vi "Set ni_measurementlink_measurement_v1_GetMetadataResponse.vi"(7 "Complete Call (T)":bool=TRUE, 8 "error in (no error)":errorcluster, 10 "package_templatemessage":T1, 11 "gRPCid":T10) -> (0 "error out":errorcluster)   [LabVIEW 2020, in "MeasurementLink Measurement Server Internal.lvlib"]
uses:
  MeasurementLink Measurement Server Internal.lvlib
  <vilib>/gRPC/LabVIEW gRPC Library/Shared/grpcId.ctl
  ni_measurementlink_measurement_v1_GetMetadataResponse.ctl
  ni_measurementlink_measurement_v1_MeasurementDetails.ctl
  ni_measurementlink_measurement_v1_MeasurementSignature.ctl
  ni_measurementlink_measurement_v1_ConfigurationParameter.ctl
  google_protobuf_Field_Kind.ctl
  ni_measurementlink_measurement_v1_ConfigurationParameter_AnnotationsEntry.ctl
  google_protobuf_Any.ctl
  ni_measurementlink_measurement_v1_Output.ctl
  ni_measurementlink_measurement_v1_UserInterfaceDetails.ctl
  ni_measurementlink_measurement_v1_GetMetadataResponse_Flat.ctl
  ni_measurementlink_measurement_v1_MeasurementDetails_Flat.ctl
  ni_measurementlink_measurement_v1_MeasurementSignature_Flat.ctl
  ni_measurementlink_measurement_v1_ConfigurationParameter_Flat.ctl
  ni_measurementlink_measurement_v1_ConfigurationParameter_AnnotationsEntry_Flat.ctl
  google_protobuf_Any_Flat.ctl
  ni_measurementlink_measurement_v1_Output_Flat.ctl
  ni_measurementlink_measurement_v1_UserInterfaceDetails_Flat.ctl
  dcc74a39-081a-4bdd-860b-8ed792803c96.vi
  RichToFlatni_measurementlink_measurement_v1_MeasurementDetails.vi
  RichToFlatni_measurementlink_measurement_v1_MeasurementSignature.vi
  RichToFlatni_measurementlink_measurement_v1_UserInterfaceDetails.vi
  <vilib>/gRPC/LabVIEW gRPC Library/Shared/TranslateGrpcError.vi
  RichToFlatni_measurementlink_measurement_v1_ConfigurationParameter.vi
  RichToFlatgoogle_protobuf_Any.vi
  RichToFlatni_measurementlink_measurement_v1_Output.vi
  RichToFlatni_measurementlink_measurement_v1_ConfigurationParameter_AnnotationsEntry.vi
  <vilib>/gRPC/LabVIEW gRPC Library/Server API/Server/Get Server DLL Path.vi
  <vilib>/Utility/error.llb/Error Cluster From Error Code.vi
  <vilib>/Utility/error.llb/Simple Error Handler.vi
  <vilib>/gRPC/LabVIEW gRPC Library/grpc-lvsupport-release.lvlib
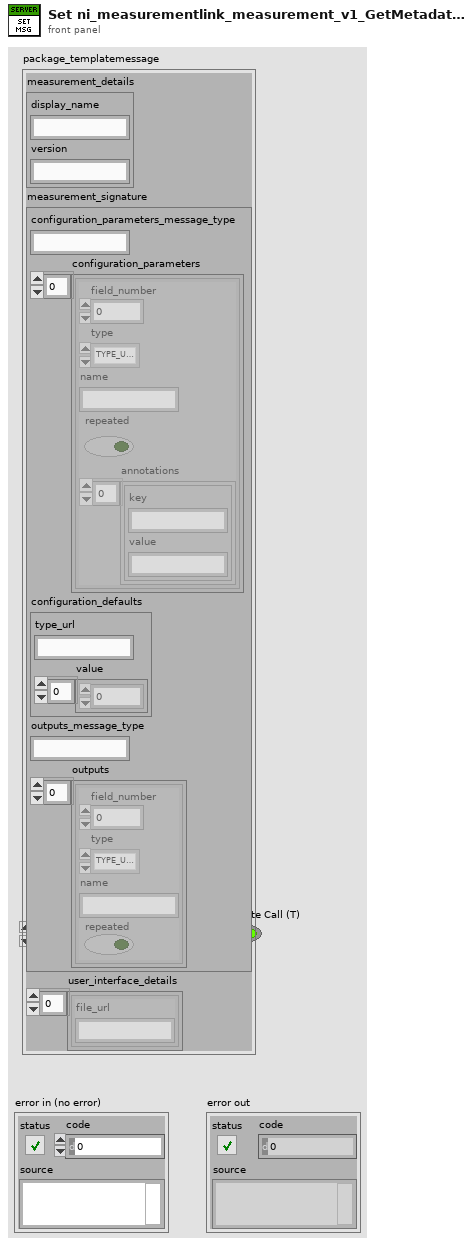
[diagram p1: front panel]
types:
  T1 = typedef "MeasurementLink Measurement Server Internal.lvlib/ni_measurementlink_measurement_v1_GetMetadataResponse.ctl" = cluster{"measurement_details":T2, "measurement_signature":T3, "user_interface_details":T9[]}
  T2 = typedef "MeasurementLink Measurement Server Internal.lvlib/ni_measurementlink_measurement_v1_MeasurementDetails.ctl" = cluster{"display_name":string, "version":string}
  T3 = typedef "MeasurementLink Measurement Server Internal.lvlib/ni_measurementlink_measurement_v1_MeasurementSignature.ctl" = cluster{"configuration_parameters_message_type":string, "configuration_parameters":T4[], "configuration_defaults":T7, "outputs_message_type":string, "outputs":T8[]}
  T4 = typedef "MeasurementLink Measurement Server Internal.lvlib/ni_measurementlink_measurement_v1_ConfigurationParameter.ctl" = cluster{"field_number":i32, "type":T5, "name":string, "repeated":bool, "annotations":T6[]}
  T5 = typedef "MeasurementLink Measurement Server Internal.lvlib/google_protobuf_Field_Kind.ctl" = enum32{"TYPE_UNKNOWN", "TYPE_DOUBLE", "TYPE_FLOAT", "TYPE_INT64", "TYPE_UINT64", "TYPE_INT32", "TYPE_FIXED64", "TYPE_FIXED32", "TYPE_BOOL", "TYPE_STRING", "TYPE_GROUP", "TYPE_MESSAGE", "TYPE_BYTES", "TYPE_UINT32", "TYPE_ENUM", "TYPE_SFIXED32", "TYPE_SFIXED64", "TYPE_SINT32", "TYPE_SINT64"}
  T6 = typedef "MeasurementLink Measurement Server Internal.lvlib/ni_measurementlink_measurement_v1_ConfigurationParameter_AnnotationsEntry.ctl" = cluster{"key":string, "value":string}
  T7 = typedef "MeasurementLink Measurement Server Internal.lvlib/google_protobuf_Any.ctl" = cluster{"type_url":string, "value":u8[]}
  T8 = typedef "MeasurementLink Measurement Server Internal.lvlib/ni_measurementlink_measurement_v1_Output.ctl" = cluster{"field_number":i32, "type":T5, "name":string, "repeated":bool}
  T9 = typedef "MeasurementLink Measurement Server Internal.lvlib/ni_measurementlink_measurement_v1_UserInterfaceDetails.ctl" = cluster{"file_url":string}
  T10 = typedef "grpc-lvsupport-release.lvlib/grpcId.ctl" = u64
  T11 = typedef "MeasurementLink Measurement Server Internal.lvlib/ni_measurementlink_measurement_v1_GetMetadataResponse_Flat.ctl" = cluster{"measurement_details":T12, "measurement_signature":T13, "user_interface_details":T18[]}
  T12 = typedef "MeasurementLink Measurement Server Internal.lvlib/ni_measurementlink_measurement_v1_MeasurementDetails_Flat.ctl" = cluster{"display_name":string, "version":string}
  T13 = typedef "MeasurementLink Measurement Server Internal.lvlib/ni_measurementlink_measurement_v1_MeasurementSignature_Flat.ctl" = cluster{"configuration_parameters_message_type":string, "configuration_parameters":T14[], "configuration_defaults":T16, "outputs_message_type":string, "outputs":T17[]}
  T14 = typedef "MeasurementLink Measurement Server Internal.lvlib/ni_measurementlink_measurement_v1_ConfigurationParameter_Flat.ctl" = cluster{"field_number":i32, "type":T5, "name":string, "repeated":bool, "annotations":T15[]}
  T15 = typedef "MeasurementLink Measurement Server Internal.lvlib/ni_measurementlink_measurement_v1_ConfigurationParameter_AnnotationsEntry_Flat.ctl" = cluster{"key":string, "value":string}
  T16 = typedef "MeasurementLink Measurement Server Internal.lvlib/google_protobuf_Any_Flat.ctl" = cluster{"type_url":string, "value":u8[]}
  T17 = typedef "MeasurementLink Measurement Server Internal.lvlib/ni_measurementlink_measurement_v1_Output_Flat.ctl" = cluster{"field_number":i32, "type":T5, "name":string, "repeated":bool}
  T18 = typedef "MeasurementLink Measurement Server Internal.lvlib/ni_measurementlink_measurement_v1_UserInterfaceDetails_Flat.ctl" = cluster{"file_url":string}
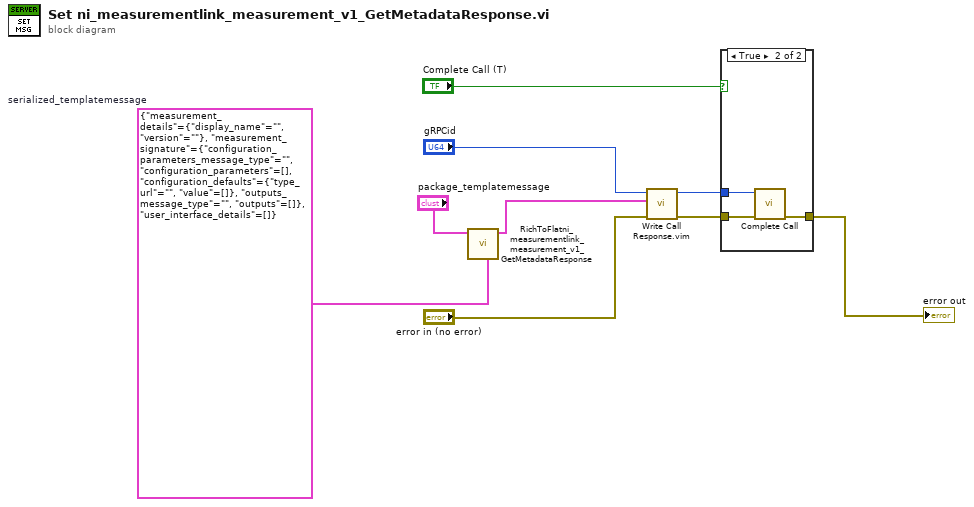
[diagram p0: block diagram]
diagram:
  w2 = T11 {"measurement_details"={"display_name"="", "version"=""}, "measurement_signature"={"configuration_parameters_message_type"="", "configuration_parameters"=[], "configuration_defaults"={"type_url"="", "value"=[]}, "outputs_message_type"="", "outputs"=[]}, "user_interface_details"=[]}  # serialized_templatemessage
  n1 = call "RichToFlatni_measurementlink_measurement_v1_GetMetadataResponse.vi"("OutputClusterType"=w2, "InputCluster"="package_templatemessage") -> ("OutputCluster"=w1:T11)  [unwired: 9 in]
  n2 = call "Write Call Response.vim"("error in"="error in (no error)", "Response Data"=w1, "gRPCid in"="gRPCid") -> ("error out"=w6:errorcluster, "gRPCid out"=w7:T10)  [unwired: 7 in]
  n3 = case shown="True" "Complete Call (T)" {
    tunnel: [w10 w13] -> w9
    tunnel: w7 -> [_ w12]
    tunnel: w6 -> [w10 w11]
    frame False {
    }
    frame True {
      n4 = call <vilib>:"Complete Call.vi"("gRPCid"=w12, "error in"=w11) -> ("error out"=w13:errorcluster)  [unwired: 8 in]
    }
  }
  "error out" <- w9
